vi "Set Mock as Parent.vi"(8 "error in (no error)":errorcluster, 11 "Mock Class Generator in":refnum<class "Responsive Mock Class Generator.lvclass">) -> (0 "error out":errorcluster, 3 "Mock Class Generator out":refnum<class "Responsive Mock Class Generator.lvclass">)   [LabVIEW 2020, in "Responsive Mock Class Generator.lvclass"]
uses:
  Responsive Mock Class Generator.lvclass
  Responsive Mock Class Generator.lvclass/Responsive Mock Class Generator.ctl
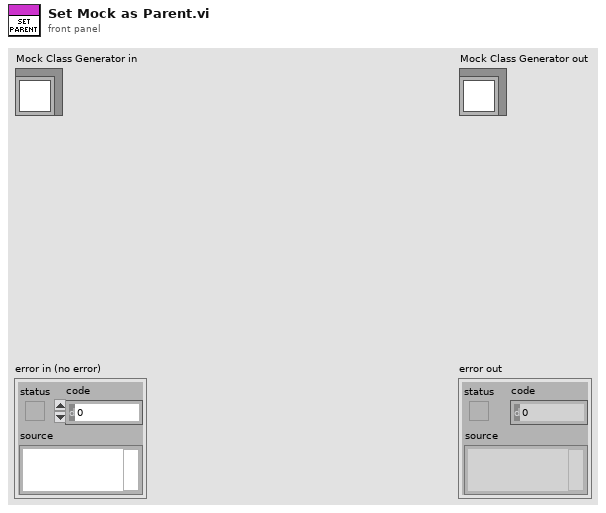
[diagram p1: front panel]
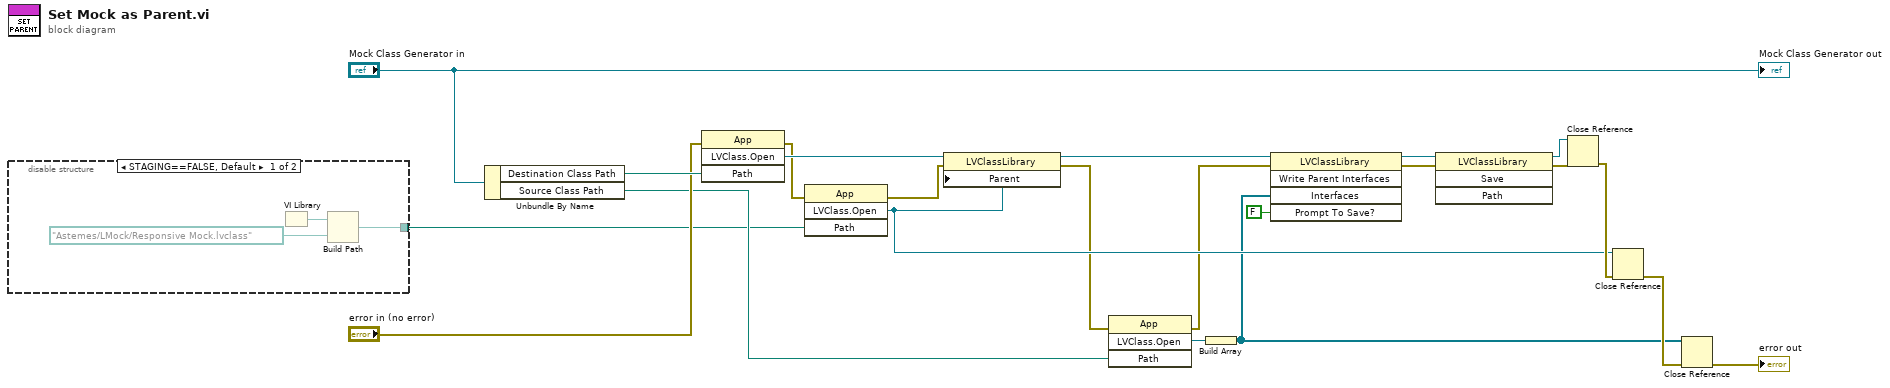
[diagram p0: block diagram]
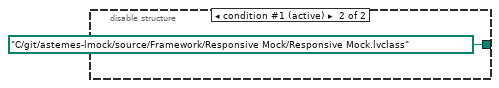
[diagram p2: hidden frame]
diagram:
  n1 = disable-structure shown="STAGING==FALSE, Default" {
    disable-tunnel: [w24 path "C:/git/astemes-lmock/source/Framework/Responsive Mock/Responsive Mock.lvclass" ("appended path")] -> w1
    frame condition #0 {
      n2 = VI Library() -> (path=w23:path)
      n3 = Build Path(base path=w23, name or relative path=path "Astemes/LMock/Responsive Mock.lvclass" ("class path")) -> (appended path=w24:path)
    }
    frame condition #1 (active) {
    }
  }
  n4 = Unbundle By Name("Mock Class Generator in") -> ("Destination Class Path"=w20:path, "Source Class Path"=w4:path)
  n5 = invoke class="App" method="LVClass.Open"(error in="error in (no error)", "Path"=w20) -> (error out=w16:errorcluster, "LVClass.Open"=w19:refnum<vi>)  [unwired: 2 in, 2 out]
  n6 = invoke class="App" method="LVClass.Open"(error in=w16, "Path"=w1) -> (error out=w22:errorcluster, "LVClass.Open"=w17:refnum<vi>)  [unwired: 2 in, 2 out]
  n7 = property class="LVClassLibrary"(reference=w19, error in=w22, "Parent"=w17) -> (reference out=w10:refnum<vi>, error out=w7:errorcluster)
  n8 = invoke class="App" method="LVClass.Open"(error in=w7, "Path"=w4) -> (error out=w6:errorcluster, "LVClass.Open"=w5:refnum<vi>)  [unwired: 2 in, 2 out]
  n9 = Build Array(w5) -> (w2:refnum<vi>[])
  n10 = invoke class="LVClassLibrary" method="Write Parent Interfaces"(reference=w10, error in=w6, "Interfaces"=w2, "Prompt To Save?"=FALSE) -> (reference out=w9:refnum<vi>, error out=w11:errorcluster)  [unwired: 1 in, 3 out]
  n11 = invoke class="LVClassLibrary" method="Save"(reference=w9, error in=w11) -> (reference out=w12:refnum<vi>, error out=w13:errorcluster)  [unwired: 2 in, 2 out]
  n12 = Close Reference(reference=w12, error in (no error)=w13) -> (error out=w18:errorcluster)
  n13 = Close Reference(reference=w17, error in (no error)=w18) -> (error out=w14:errorcluster)
  n14 = Close Reference(reference=w2, error in (no error)=w14) -> (error out=→"error out":errorcluster)
  "Mock Class Generator out" <- "Mock Class Generator in"
